vi "DefineScan.vi"(5 "tc":dbl, 7 "dt (in tc)":u32, 10 "DimensionScans":cluster{"Start":dbl, "Stop":dbl, "Steps":u32}[](array[cluster]), 11 "Dimensions":u16[](array[ring]) items=["X", "Y", "Z"]) -> (0 "Scans":cluster{"Start":dbl, "Stop":dbl, "Steps":u32}[](array[cluster]), 1 "ScanDim":string[](array[string]), 2 "Dim3Strings":string[](array[string]), 3 "Dim2Strings":string[](array[string]), 4 "ScanArray":dbl[][][](array[numeric]), 6 "Estimated Time (ms)":dbl)   [LabVIEW 2013]
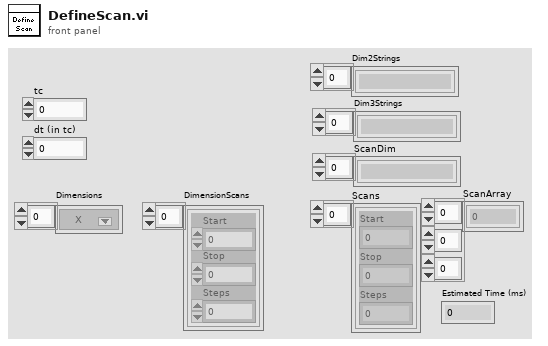
[diagram p1: front panel]
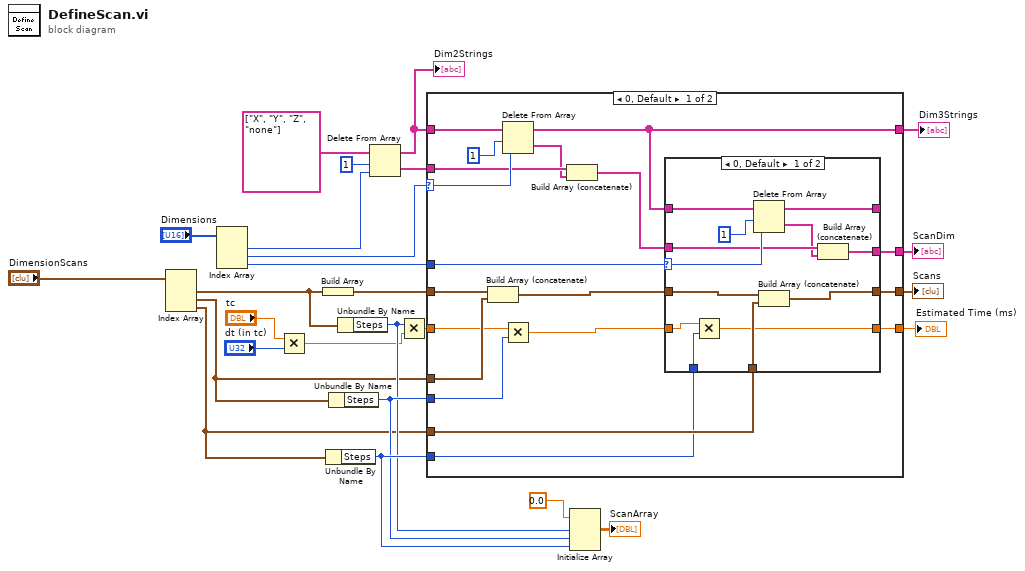
[diagram p0: block diagram]
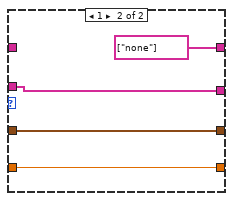
[diagram p2: hidden frame]
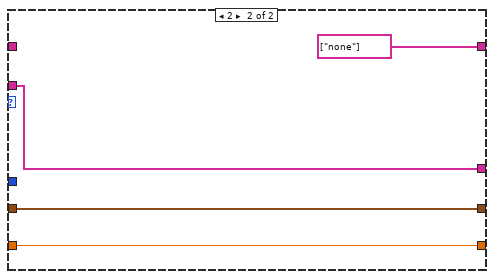
[diagram p3: hidden frame]
diagram:
  n1 = Index Array(array="DimensionScans") -> (element #1=w3:cluster{"Start":dbl, "Stop":dbl, "Steps":u32}, element #2=w1:cluster{"Start":dbl, "Stop":dbl, "Steps":u32}, element #3=w2:cluster{"Start":dbl, "Stop":dbl, "Steps":u32})  [unwired: 3 in]
  n2 = Index Array(array="Dimensions") -> (element #1=w7:u16, element #2=w6:u16, element #3=w5:u16)  [unwired: 3 in]
  n3 = Multiply(x="tc", y="dt (in tc)") -> (x*y=w21:dbl)
  n4 = Build Array(w3) -> (w16:cluster{"Start":dbl, "Stop":dbl, "Steps":u32}[])
  n5 = Unbundle By Name(w2) -> ("Steps"=w25:u32)
  n6 = Unbundle By Name(w1) -> ("Steps"=w24:u32)
  n7 = Unbundle By Name(w3) -> ("Steps"=w23:u32)
  n8 = Delete From Array(array=string[] ["X", "Y", "Z", "none"], length=1, index=w7) -> (deleted portion=w14:string[], array with subset deleted=w13:string[])
  "Dim2Strings" <- w13
  n9 = Multiply(x=w23, y=w21) -> (x*y=w17:dbl)
  n10 = case shown="0, Default" w6 {
    selector: w6 -> [w44 _]
    tunnel: [w39 string[] ["none"] ("Strings []")] -> w15
    tunnel: w13 -> [w43 _]
    tunnel: w14 -> [w42 w65]
    tunnel: [w38 w65] -> w19
    tunnel: w16 -> [w37 w64]
    tunnel: [w33 w64] -> w20
    tunnel: w1 -> [w36 _]
    tunnel: w2 -> [w34 _]
    tunnel: w17 -> [w32 w63]
    tunnel: [w28 w63] -> w18
    tunnel: w24 -> [w31 _]
    tunnel: w25 -> [w29 _]
    tunnel: w5 -> [w27 _]
    frame 0, Default {
      n11 = Build Array (concatenate)(w37, w36) -> (w35:cluster{"Start":dbl, "Stop":dbl, "Steps":u32}[])
      n12 = Delete From Array(array=w43, length=1, index=w44) -> (deleted portion=w41:string[], array with subset deleted=w39:string[])
      n13 = Multiply(x=w32, y=w31) -> (x*y=w30:dbl)
      n14 = Build Array (concatenate)(w42, w41) -> (w40:string[])
      n15 = case shown="0, Default" w27 {
        selector: w27 -> [w57 _]
        tunnel: [w53 string[] ["none"] ("Strings []")] -> _
        tunnel: w40 -> [w56 w61]
        tunnel: [w55 w61] -> w38
        tunnel: w39 -> [w54 _]
        tunnel: w35 -> [w51 w60]
        tunnel: w34 -> [w50 _]
        tunnel: [w49 w60] -> w33
        tunnel: w30 -> [w48 w59]
        tunnel: w29 -> [w47 _]
        tunnel: [w46 w59] -> w28
        frame 0, Default {
          n16 = Multiply(x=w48, y=w47) -> (x*y=w46:dbl)
          n17 = Delete From Array(array=w54, length=1, index=w57) -> (deleted portion=w52:string[], array with subset deleted=w53:string[])
          n18 = Build Array (concatenate)(w51, w50) -> (w49:cluster{"Start":dbl, "Stop":dbl, "Steps":u32}[])
          n19 = Build Array (concatenate)(w56, w52) -> (w55:string[])
        }
        frame 1 {
        }
      }
    }
    frame 2 {
    }
  }
  "Estimated Time (ms)" <- w18
  "Dim3Strings" <- w15
  "ScanDim" <- w19
  "Scans" <- w20
  n20 = Initialize Array(0.0, w23, w24, w25) -> (→"ScanArray":dbl[][][])
